vi "FTW-ERR-Assert-AbstractMethodCall.vi"(11 "error in":errorcluster) -> (15 "error out":errorcluster)   [LabVIEW 2013]
doc: "Toto, I've a feeling we're not in Kansas any more.... We must be over the rainbow!"
uses:
  FTW-ERR-ThrowError.vi
panel:
  # "Inputs"
  # "Outputs"
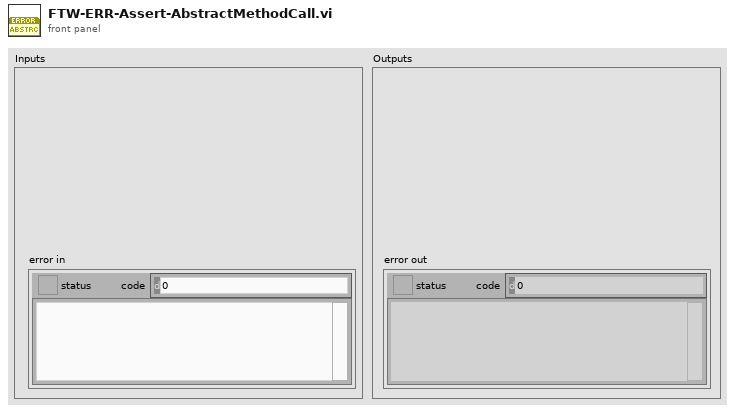
[diagram p1: front panel]
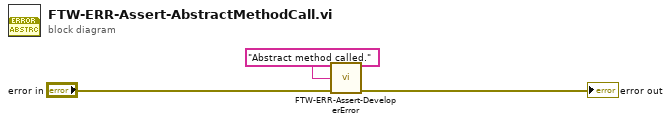
[diagram p0: block diagram]
diagram:
  n1 = call "FTW-ERR-Assert-DeveloperError.vi"("Reason this error should never happen"="Abstract method called.", "error in"="error in") -> ("error out"=→"error out":errorcluster)  [unwired: 13 in]
